vi "HW_Get_data_flow_from_serial_port.vi"(6 "error in":errorcluster, 8 "VISA resource name in":refnum<visa-resource-name>) -> (0 "Not empty?":bool, 1 "error out":errorcluster, 2 "Timestamp":timestamp, 3 "Data":string, 5 "VISA resource name out":refnum<visa-resource-name>)   [LabVIEW 2018, in "Tracker.lvlib"]
uses:
  Tracker.lvlib
  <vilib>/Instr/_visa.llb/Select Event Type.ctl
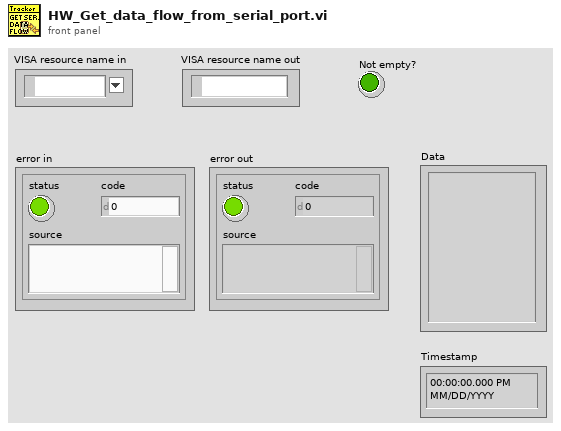
[diagram p1: front panel]
types:
  T1 = typedef "Select Event Type.ctl" = u32
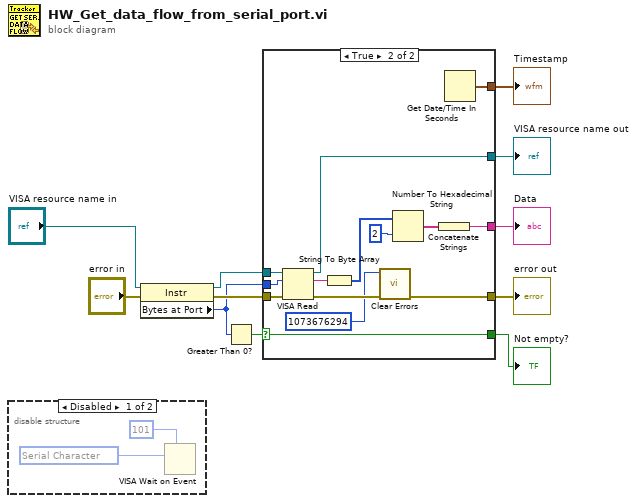
[diagram p0: block diagram]
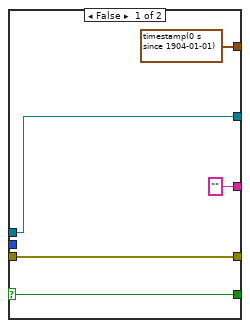
[diagram p3: hidden frame]
diagram:
  n1 = disable-structure shown="Disabled" {
    frame Disabled {
      w13 = T1 1073684533 items=["Service Request"=1073684491, "Trigger"=3221168138, "Clear"=1073684493, "VXI Signal"=1073684512, "VXI/VME Interrupt"=3221168161, "VXI/VME Sysfail"=1073684509, "VXI/VME Sysreset"=1073684510, "GPIB CIC"=1073684498, "GPIB Talk"=1073684499, "GPIB Listen"=1073684500, "PXI Interrupt"=1073684514, "Serial Break"=1073684515, "Serial TermChar"=1073684516, "Serial CTS"=1073684521, "Serial DSR"=1073684522, "Serial DCD"=1073684524, "Serial RI"=1073684526, "Serial Character"=1073684533, "USB Interrupt"=1073684535, "All Enabled"=1073709055] ("Event Type")
      n2 = VISA Wait on Event(7:u32 101 ("timeout (0)"), 10:w13) -> ()  [unwired: 3 in, 4 out]
    }
    frame Enabled {
    }
  }
  n3 = property class="Instr"(reference="VISA resource name in", error in="error in") -> (reference out=w10:refnum<visa-resource-name>, error out=w11:errorcluster, "Bytes at Port"=w9:u32)
  n4 = Greater Than 0?(x=w9) -> (x > 0?=w8:bool)
  n5 = case shown="True" w8 {
    selector: w8 -> [w17 w22]
    tunnel: [w18 w30] -> w7
    tunnel: w9 -> [_ w29]
    tunnel: w11 -> [w14 w28]
    tunnel: w10 -> [w18 w27]
    tunnel: [w17 w22] -> w6
    tunnel: ["" w21] -> w5
    tunnel: [timestamp(0 s since 1904-01-01) ("seconds since 1Jan1904") w20] -> w4
    tunnel: [w14 w19] -> w3
    frame False {
    }
    frame True {
      n6 = VISA Read(VISA resource name=w27, byte count=w29, error in (no error)=w28) -> (VISA resource name out=w30:refnum<visa-resource-name>, read buffer=w31:string, error out=w32:errorcluster)  [unwired: 1 out]
      n7 = String To Byte Array(string=w31) -> (unsigned byte array=w23:u8[])
      n8 = call <vilib>:"Clear Errors.vi"("error in (no error)"=w32, "specific error code to clear (0: all)"=1073676294) -> ("error out"=w19:errorcluster)  [unwired: 4 in, 1 out]
      n9 = Number To Hexadecimal String(1:i16 2 ("width (-)"), 2:w23) -> (0:w25:string[])
      n10 = Concatenate Strings(w25) -> (w21:string)
      n11 = Get Date/Time In Seconds ("Current time")() -> (seconds since 1Jan1904=w20:timestamp)
    }
  }
  "VISA resource name out" <- w7
  "Not empty?" <- w6
  "Data" <- w5
  "Timestamp" <- w4
  "error out" <- w3
